vi "tvac_gui_v1.vi"() -> ()   [LabVIEW 2017]
uses:
  <vilib>/httpClient/ClientHandle.ctl
  <vilib>/httpClient/POSTBuffer.vi
  <vilib>/httpClient/LabVIEWHTTPClient.lvlib
panel:
  out "body 2":string
  in  "Tab Control":T1(tab)
  in  "TC Graph 2":T2
  out "TC Display":T3
  out "Waveform Chart":waveform(dbl)[](graph)=[{"t0"=timestamp(3580757854.087 s since 1904-01-01), "dt"=1.0, "Y"=[750.0616827041697]}, {"t0"=timestamp(3580757854.087 s since 1904-01-01), "dt"=1.0, "Y"=[750.0616827041697]}, {"t0"=timestamp(3580757854.087 s since 1904-01-01), "dt"=1.0, "Y"=[750.0616827041697]}]
  out "body":string
  in  "stop":bool
  in  "Cluster":T4 {"Zone 1"."average" items=["Average", "Maximum", "Minimum"]; "Zone 2"."average" items=["Average", "Maximum", "Minimum"]}
  in  "Run 4":bool
  in  "Run 3":bool
  in  "Run 2":bool
  in  "Run":bool
  out "body 3":string
  out "JSON string":string
  out "Custom Graphs 4":dbl[](graph)
  out "Custom Graphs 3":dbl[](graph)
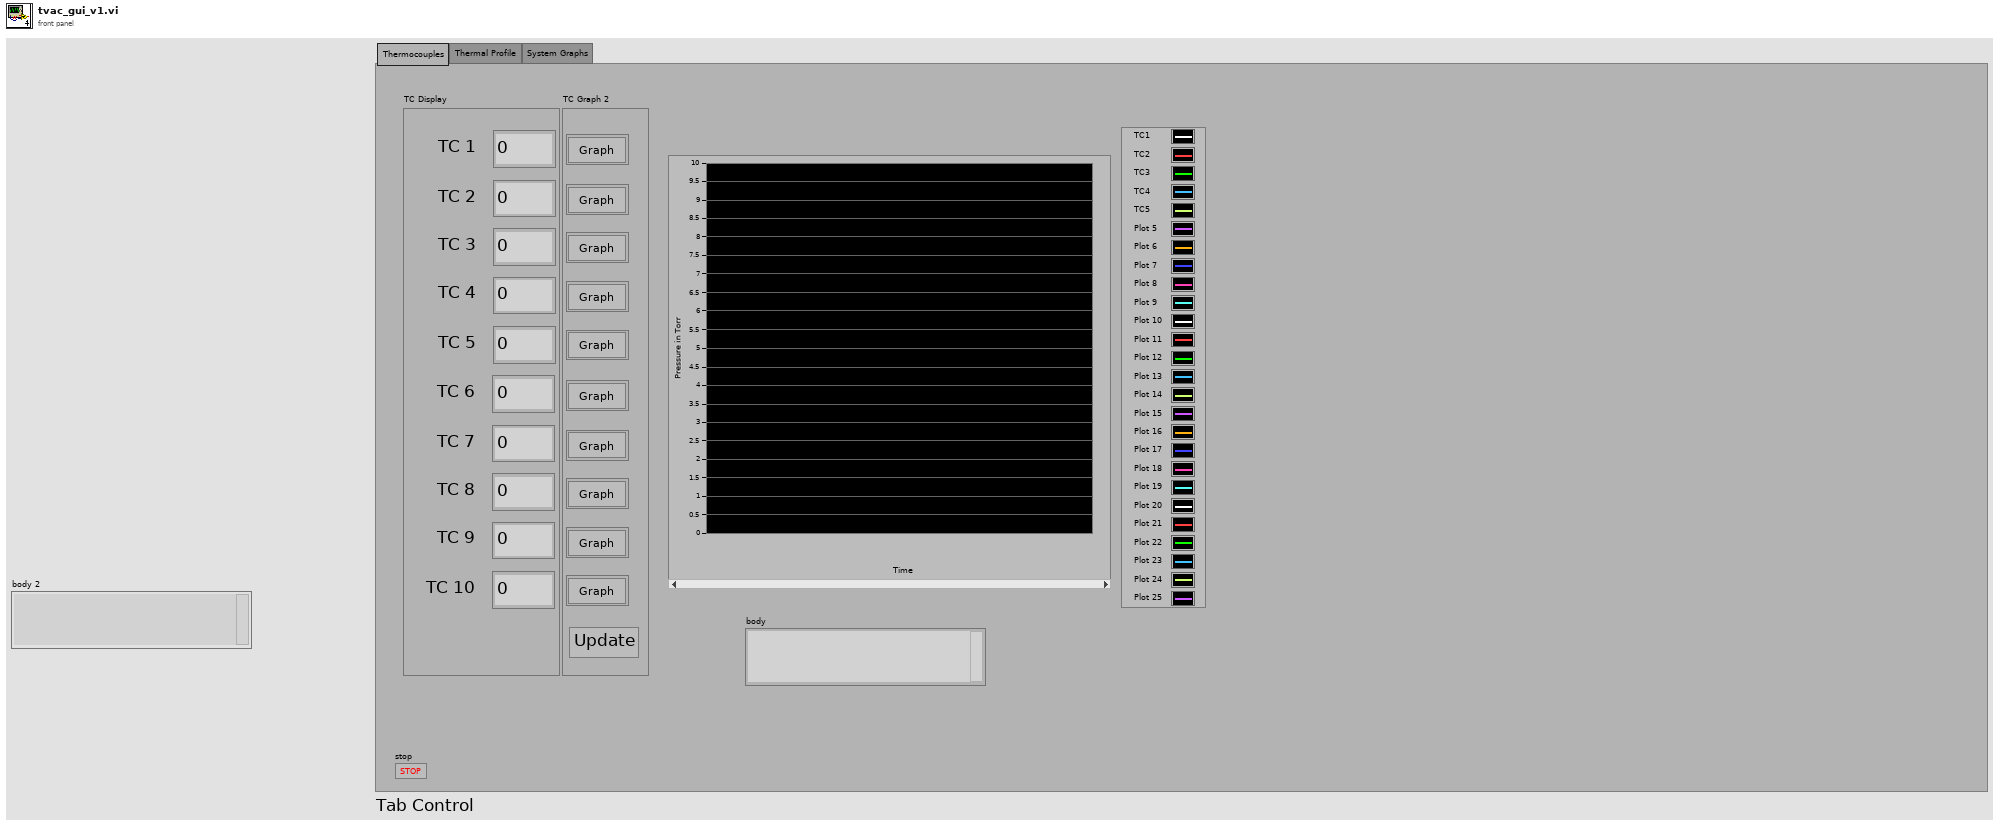
[diagram p1: front panel]
types:
  T1 = enum32{"Thermocouples", "Thermal Profile", "System Graphs"}
  T2 = cluster{"TC 1":bool, "TC 2":bool, "TC 3":bool, "TC 4":bool, "TC 5":bool, "TC 6":bool, "TC 7":bool, "TC 8":bool, "TC 9":bool, "TC 10":bool, "Update":bool}
  T3 = cluster{"TC 1":dbl, "TC 2":dbl, "TC 3":dbl, "TC 4":dbl, "TC 5":dbl, "TC 6":dbl, "TC 7":dbl, "TC 8":dbl, "TC 9":dbl, "TC 10":dbl}
  T4 = cluster{"Zone 2":cluster{"zone":dbl, "average":u16, "thermalprofile":cluster{"thermalsetpoint":dbl, "tempgoal":dbl, "ramp":dbl, "soakduration":dbl}, "thermocouples":dbl[]}, "Zone 1":cluster{"zone":dbl, "average":u16, "thermalprofile":cluster{"thermalsetpoint":dbl, "tempgoal":dbl, "ramp":dbl, "soakduration":dbl}, "thermocouples":dbl[]}}
  T5 = typedef "LabVIEWHTTPClient.lvlib/ClientHandle.ctl" = refnum<k1>
  T6 = cluster{"go":bool, "Http session":T5, "URL prefex":string}
  T7 = cluster{"time":string, "tcs":cluster{"thermocouple":i32, "time":i32, "temp":i32, "working":i32}[]}
  T8 = cluster{"thermocouple":i32, "time":i32, "temp":i32, "working":i32}[]
  T9 = cluster{"thermocouple":i32, "time":i32, "temp":i32, "working":i32}
  T10 = cluster{"zone":i32, "profileuuid":string, "average":i32, "zoneUUID":string, "termalprofiles":cluster{"termalsetpoint":i32, "tempgoal":i32, "temp":i32, "soakduration":i32, "duration":i32, "ramp":i32}[], "thermocouples":cluster{"thermocouple":i32, "time":i32, "temp":i32, "working":string}[]}
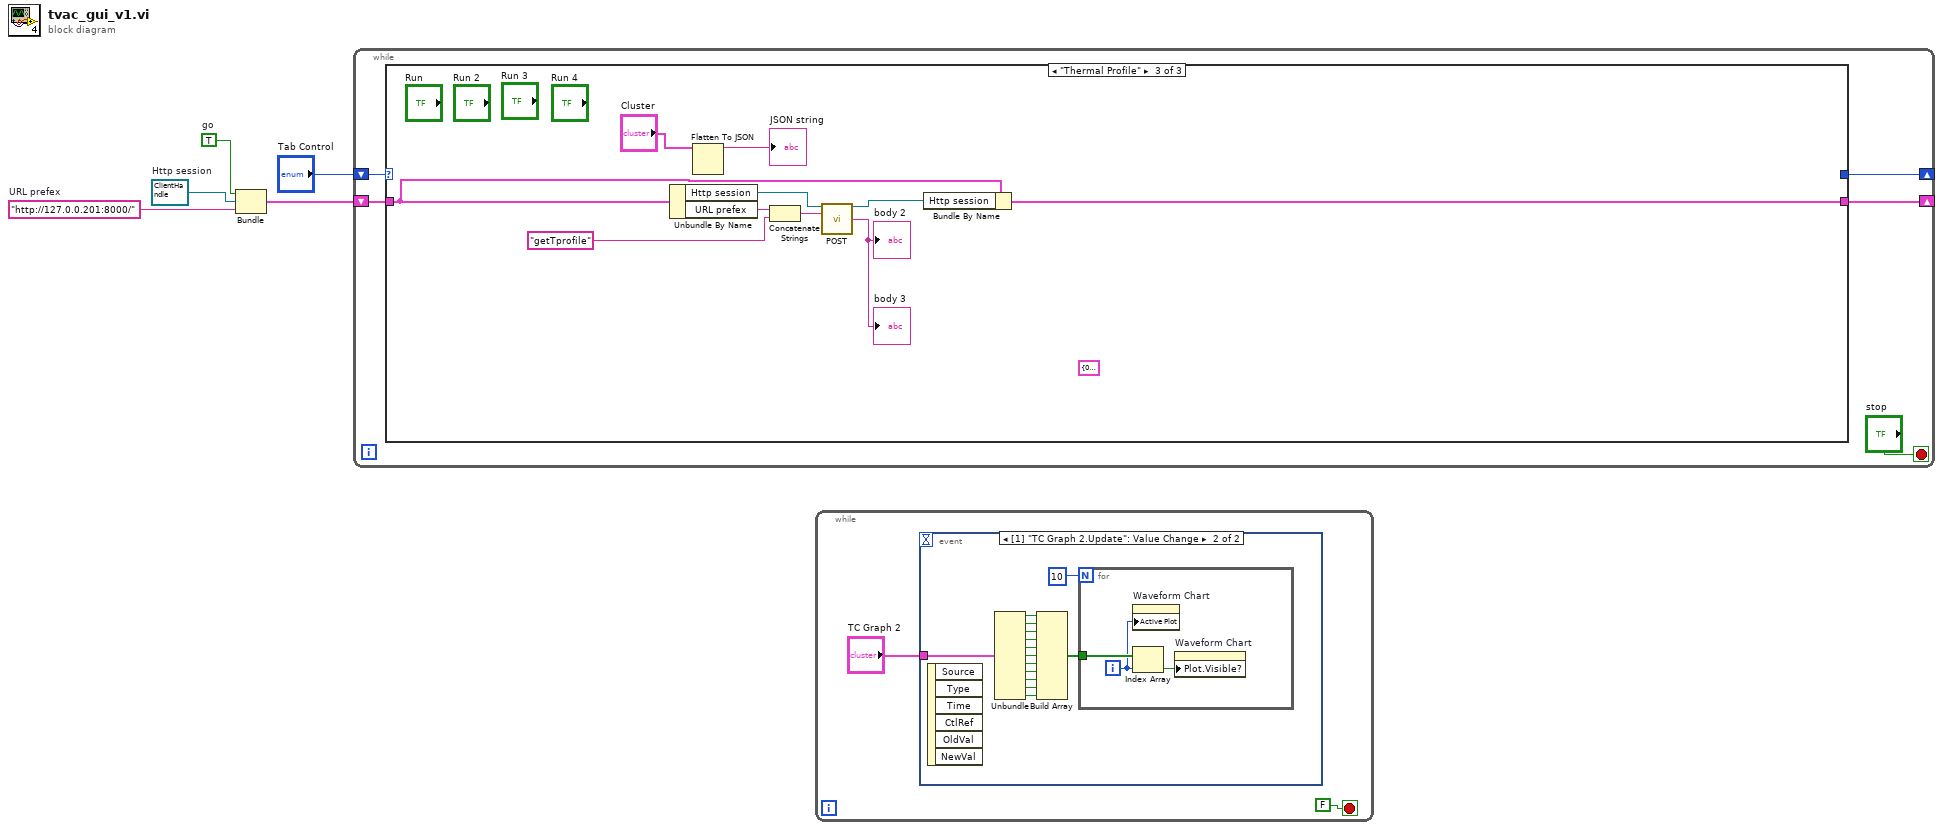
[diagram p0: block diagram]
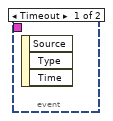
[diagram p2: hidden frame]
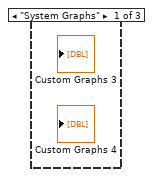
[diagram p3: hidden frame]
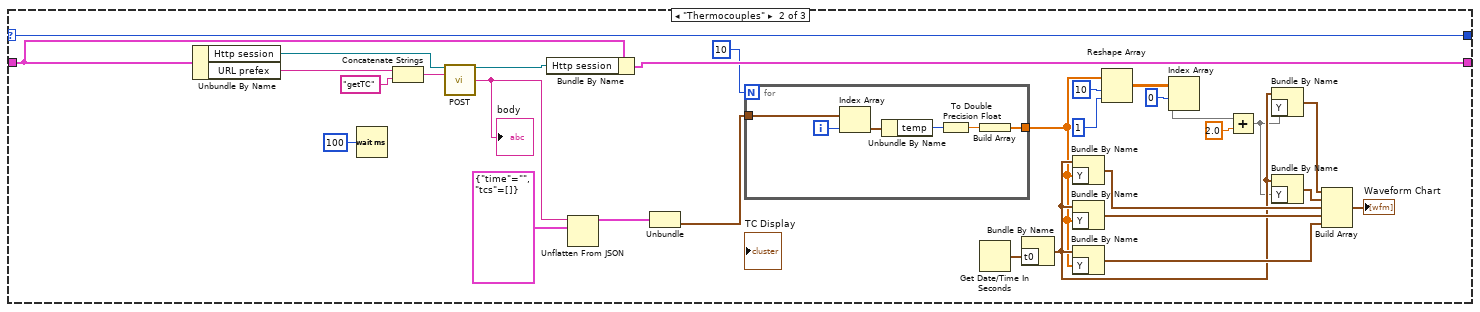
[diagram p4: hidden frame]
diagram:
  w3 = "http://127.0.0.201:8000/"  # URL prefex
  w4 = T5 refnum  # Http session
  w5 = TRUE  # go
  n1 = Bundle("go"=w5, "Http session"=w4, "URL prefex"=w3) -> (w2:T6)  [unwired: 1 in]
  n2 = while {
    shift-right: [w9] -> _
    shift-left: w2 -> [w10]
    shift-right: [w7] -> _
    shift-left: "Tab Control" -> [w8]
    stop <- "stop" stop-if-true
    n3 = case shown="\"Thermal Profile\"" w8 {
      selector: w8 -> [_ w12 _]
      tunnel: w10 -> [_ w24 w49]
      tunnel: [_ w23 w50] -> w9
      tunnel: [_ w12 _] -> w7
      frame "System Graphs" {
      }
      frame "Thermocouples" {
        n4 = Unbundle By Name(w24) -> ("Http session"=w32:T5, "URL prefex"=w30:string)
        n5 = Wait (ms)(milliseconds to wait=u32 100) -> ()  [unwired: 1 out]
        n6 = Concatenate Strings(w30, "getTC" ("url")) -> (w31:string)
        n7 = call-poly <vilib>:"POST.vi"("client handle"=w32, "url"=w31) -> ("client handle out"=w25:T5, "body"=w27:string)  [unwired: 10 in, 2 out]
        "body" <- w27
        n8 = Bundle By Name(cluster=w24, "Http session"=w25) -> (w23:T6)
        n9 = Unflatten From JSON(JSON string=w27, type and defaults=T7 {"time"="", "tcs"=[]}) -> (value=w26:T7)  [unwired: 5 in, 1 out]
        n10 = Unbundle(w26) -> ("tcs"=w22:T8)  [unwired: 1 out]
        n11 = for {
          N: 10 -> [_]
          tunnel: w22 -> [w46]
          tunnel: [w41] -> w20
          i -> [w45]
          n12 = Index Array(array=w46, index=w45) -> (element=w44:T9)
          n13 = Unbundle By Name(w44) -> ("temp"=w43:i32)
          n14 = To Double Precision Float(number=w43) -> (double precision float=w42:dbl)
          n15 = Build Array(w42) -> (w41:dbl[])
        }
        n16 = Get Date/Time In Seconds() -> (seconds since 1Jan1904=w40:timestamp)
        n17 = Bundle By Name("t0"=w40) -> (w33:waveform(dbl))  [unwired: 1 in]
        n18 = Bundle By Name(cluster=w33, "Y"=w20) -> (w37:waveform(dbl))
        n19 = Bundle By Name(cluster=w33, "Y"=w20) -> (w35:waveform(dbl))
        n20 = Bundle By Name(cluster=w33, "Y"=w20) -> (w34:waveform(dbl))
        n21 = Reshape Array(w20, 10 ("dimension size"), 1 ("dimension size")) -> (w17:dbl[][])
        n22 = Index Array(array=w17, index (row)=0) -> (element=w14:dbl[])  [unwired: 1 in]
        n23 = Add(x=w14, y=2.0) -> (x+y=w13:dbl[])
        n24 = Bundle By Name(cluster=w33, "Y"=w13) -> (w39:waveform(dbl))
        n25 = Bundle By Name(cluster=w33, "Y"=w13) -> (w38:waveform(dbl))
        n26 = Build Array(w39, w38, w37, w35, w34) -> (→"Waveform Chart":waveform(dbl)[])
      }
      frame "Thermal Profile" {
        (unwired) T10 {"zone"=0, "profileuuid"="", "average"=0, "zoneUUID"="", "termalprofiles"=[], "thermocouples"=[]}
        n27 = Unbundle By Name(w49) -> ("Http session"=w56:T5, "URL prefex"=w54:string)
        n28 = Flatten To JSON(anything="Cluster") -> (JSON string=→"JSON string":string)  [unwired: 2 in, 1 out]
        n29 = Concatenate Strings(w54, "getTprofile" ("url")) -> (w55:string)
        n30 = call-poly <vilib>:"POST.vi"("client handle"=w56, "url"=w55) -> ("client handle out"=w51:T5, "body"=→"body 2" →"body 3":string)  [unwired: 10 in, 2 out]
        n31 = Bundle By Name(cluster=w49, "Http session"=w51) -> (w50:T6)
      }
    }
  }
  n32 = while {
    stop <- FALSE stop-if-true
    n33 = event shown="[1] \"TC Graph 2.Update\": Value Change" {
      selector: _ -> [_ _]
      dyn-events: _ -> [_ _]
      timeout: _ -> [_ _]
      tunnel: "TC Graph 2" -> [_ w72]
      event Timeout {
        n34 = event-data() -> ()  [unwired: 1 in, 3 out]
      }
      event "TC Graph 2.Update": Value Change {
        n35 = event-data() -> ()  [unwired: 1 in, 6 out]
        n36 = Unbundle(w72) -> ("TC 1"=w71:bool, "TC 2"=w70:bool, "TC 3"=w69:bool, "TC 4"=w68:bool, "TC 5"=w67:bool, "TC 6"=w64:bool, "TC 7"=w63:bool, "TC 8"=w62:bool, "TC 9"=w61:bool, "TC 10"=w60:bool, "Update"=w59:bool)
        n37 = Build Array(w71, w70, w69, w68, w67, w64, w63, w62, w61, w60, w59) -> (w66:bool[])
        n38 = for {
          N: 10 -> [_]
          tunnel: w66 -> [w75]
          i -> [w74]
          n39 = property on="Waveform Chart" class="WFChart (strict)"("Active Plot"=w74) -> ()  [unwired: 2 in, 2 out]
          n40 = Index Array(array=w75, index=w74) -> (element=w73:bool)
          n41 = property on="Waveform Chart" class="WFChart (strict)"("Plot.Visible?"=w73) -> ()  [unwired: 2 in, 2 out]
        }
      }
    }
  }
